vi "Intensity integral.vi"(1 "width":i32, 2 "begin":i32, 3 "数组":dbl[][](array[numeric])) -> (0 "数组 2":dbl[](array[numeric]))   [LabVIEW 2018]
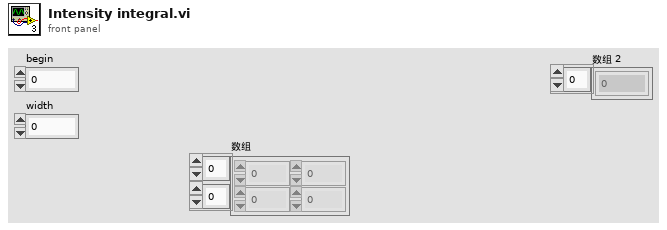
[diagram p1: front panel]
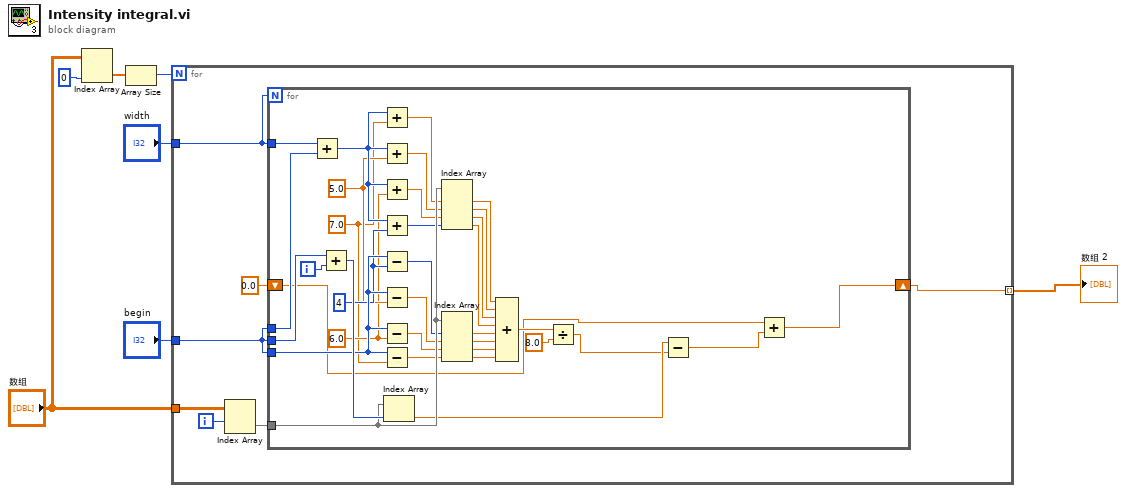
[diagram p0: block diagram]
diagram:
  n1 = Index Array(array="数组", index (col)=0 ("禁用的索引 (列)")) -> (element=w5:dbl[])  [unwired: 1 in]
  n2 = Array Size(array=w5) -> (size(s)=w2:i32)
  n3 = for {
    N: w2 -> [_]
    tunnel: "数组" -> [w14]
    tunnel: "begin" -> [w10]
    tunnel: "width" -> [w11]
    tunnel: [w8] -> w1 mode=indexing
    i -> [w13]
    n4 = Index Array(array=w14, index (row)=w13) -> (element=w12:dbl[])  [unwired: 1 in]
    n5 = for {
      N: w11 -> [_]
      tunnel: w12 -> [w46]
      tunnel: w10 -> [w48]
      tunnel: w10 -> [w41]
      tunnel: w11 -> [w40]
      tunnel: w10 -> [w39]
      shift-right: [w16] -> w8
      shift-left: 0.0 -> [w15]
      i -> [w49]
      w30 = 7.0 ("y")
      w31 = 6.0 ("y")
      w32 = 5.0 ("y")
      w33 = 4 ("y")
      n6 = Add(x=w40, y=w39) -> (x+y=w36:i32)
      n7 = Add(x=w48, y=w49) -> (x+y=w47:i32)
      n8 = Add(x=w36, y=w30) -> (x+y=w38:dbl)
      n9 = Add(x=w36, y=w32) -> (x+y=w37:dbl)
      n10 = Add(x=w36, y=w31) -> (x+y=w35:dbl)
      n11 = Add(x=w36, y=w33) -> (x+y=w34:i32)
      n12 = Subtract(x=w41, y=w33) -> (x-y=w45:i32)
      n13 = Subtract(x=w41, y=w32) -> (x-y=w44:dbl)
      n14 = Subtract(x=w41, y=w31) -> (x-y=w43:dbl)
      n15 = Subtract(x=w41, y=w30) -> (x-y=w42:dbl)
      n16 = Index Array(array=w46, index=w47) -> (element=w19:dbl)
      n17 = Index Array(array=w46, index #1=w38, index #2=w37, index #3=w35, index #4=w34) -> (element #1=w29:dbl, element #2=w28:dbl, element #3=w27:dbl, element #4=w26:dbl)
      n18 = Index Array(array=w46, index #1=w45, index #2=w44, index #3=w43, index #4=w42) -> (element #1=w25:dbl, element #2=w24:dbl, element #3=w23:dbl, element #4=w22:dbl)
      n19 = Compound Arithmetic op=unknown(w29, w28, w27, w26, w25, w24, w23, w22) -> (w21:dbl)
      n20 = Divide(x=w21, y=8.0) -> (x/y=w18:dbl)
      n21 = Subtract(x=w19, y=w18) -> (x-y=w17:dbl)
      n22 = Add(x=w15, y=w17) -> (x+y=w16:dbl)
    }
  }
  "数组 2" <- w1
